vi "Get MetaData from Configurations.vi"(8 "error in":errorcluster, 10 "Measurement":refnum<class "MeasurementService.lvclass">, 11 "Configuration Cluster":variant) -> (0 "error out":errorcluster, 3 "configuration_parameters":T1[](array[typedef]))   [LabVIEW 2020, in "MeasurementLink Measurement Server.lvlib"]
uses:
  MeasurementLink Measurement Server.lvlib
  MeasurementLink Measurement Server Internal/RPC Messages/ni_measurementlink_measurement_v1_ConfigurationParameter.ctl
  MeasurementLink Measurement Server Internal/RPC Messages/ni_measurementlink_measurement_v1_ConfigurationParameter_AnnotationsEntry.ctl
  <vilib>/Utility/Data Type/NI_Data Type.lvlib
  MeasurementLink Measurement Server Internal/MeasurementLink Measurement Server Internal.lvlib
  RPC Service/MeasurementService/MeasurementService.lvclass
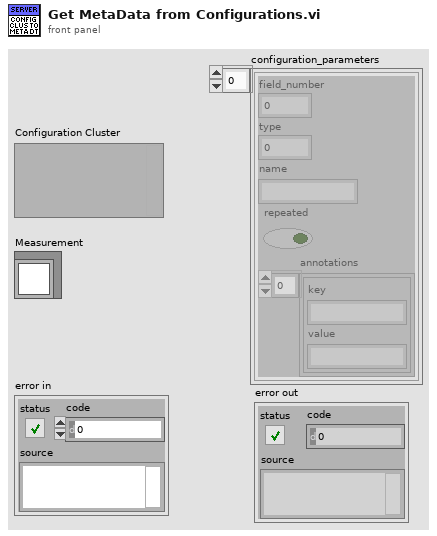
[diagram p1: front panel]
types:
  T1 = typedef "MeasurementLink Measurement Server Internal.lvlib/ni_measurementlink_measurement_v1_ConfigurationParameter.ctl" = cluster{"field_number":i32, "type":i32, "name":string, "repeated":bool, "annotations":T2[]}
  T2 = typedef "MeasurementLink Measurement Server Internal.lvlib/ni_measurementlink_measurement_v1_ConfigurationParameter_AnnotationsEntry.ctl" = cluster{"key":string, "value":string}
  T3 = cluster{"Parameter Name":string, "Annotations":cluster{"key":string, "value":string}[]}[]
  T4 = typedef "NI_Data Type.lvlib/Data Type.ctl" = enum8{"Invalid Type", "Void", "I8", "I16", "I32", "I64", "U8", "U16", "U32", "U64", "Single Float", "Double Float", "Extended Float", "Single Complex", "Double Complex", "Extended Complex", "Enum U8", "Enum U16", "Enum U32", "Enum U64", "Single Float With Unit", "Double Float With Unit", "Extended Float With Unit", "Single Complex with Unit", "Double Complex with Unit", "Extended Complex with Unit", "Boolean", "String", "Path", "Picture", "Tag", "Array", "Cluster", "Variant", "LV Variant", "Waveform", "Timestamp", "Digital Waveform", "Digital Data", "ExpressData", "Refnum", "External Data", "VI", "Poly VI", "LabVIEW Class Instance", "Fixed Point", "Set Collection", "Map Collection"}
  T5 = typedef "MeasurementLink Measurement Server.lvlib/google_protobuf_Field_Kind.ctl" = enum32{"TYPE_UNKNOWN", "TYPE_DOUBLE", "TYPE_FLOAT", "TYPE_INT64", "TYPE_UINT64", "TYPE_INT32", "TYPE_FIXED64", "TYPE_FIXED32", "TYPE_BOOL", "TYPE_STRING", "TYPE_GROUP", "TYPE_MESSAGE", "TYPE_BYTES", "TYPE_UINT32", "TYPE_ENUM", "TYPE_SFIXED32", "TYPE_SFIXED64", "TYPE_SINT32", "TYPE_SINT64"}
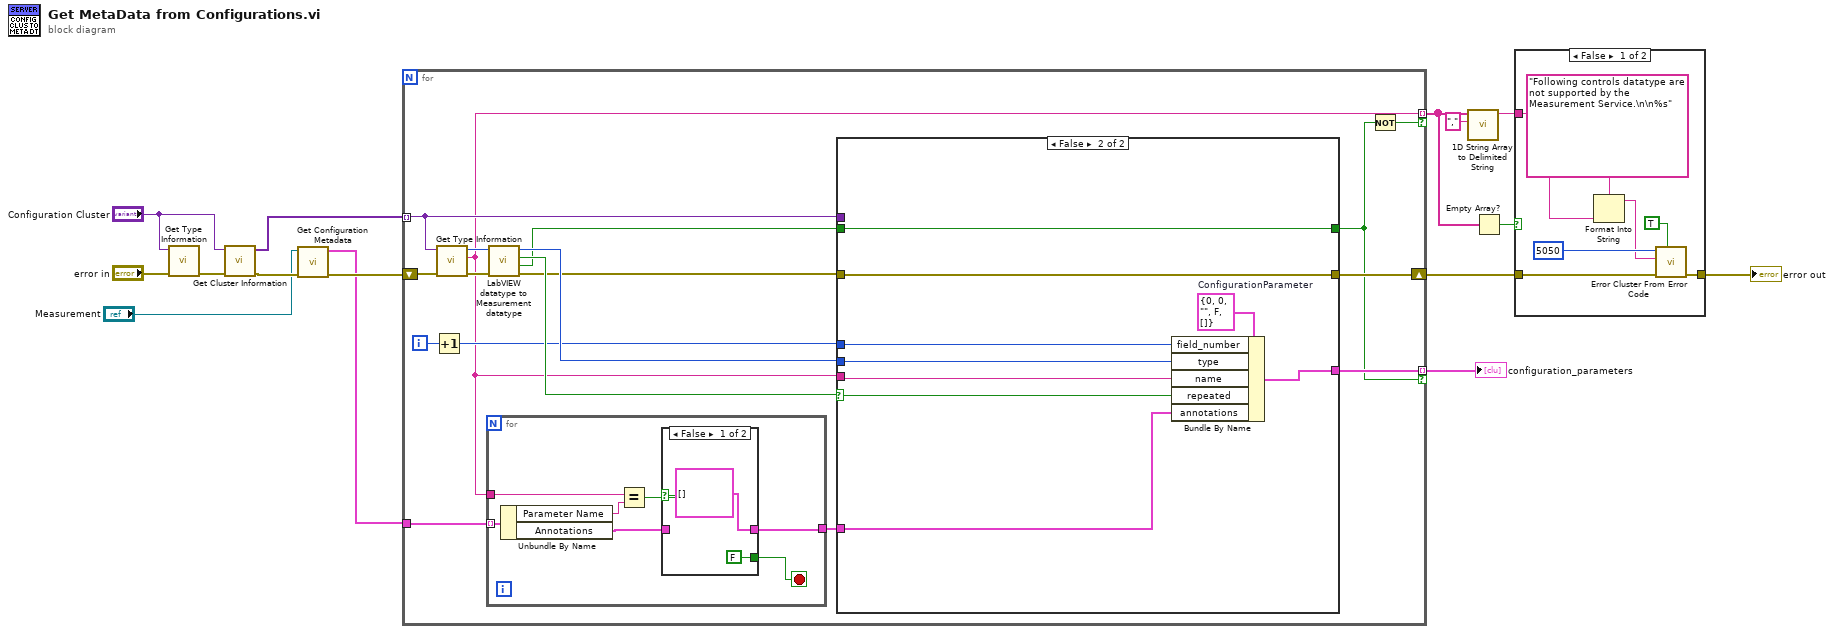
[diagram p0: block diagram]
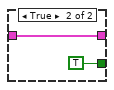
[diagram p3: hidden frame]
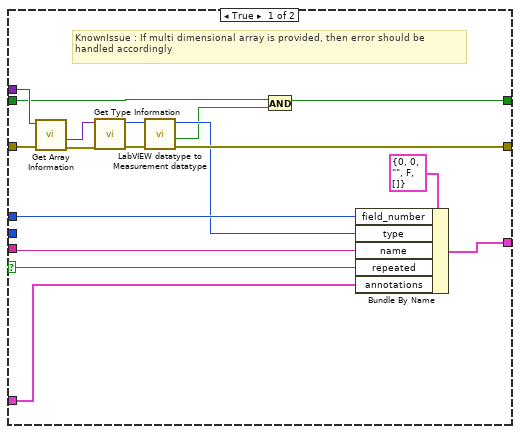
[diagram p4: hidden frame]
diagram:
  n1 = call <vilib>:"Get Type Information.vi"("error in (no error)"="error in", "variant"="Configuration Cluster") -> ("error out"=w15:errorcluster)  [unwired: 5 in, 4 out]
  n2 = call <vilib>:"Get Cluster Information.vi"("error in (no error)"=w15, "variant"="Configuration Cluster") -> ("error out"=w4:errorcluster, "cluster elements"=w14:variant[])  [unwired: 8 in]
  n3 = call "Get Configuration Metadata.vi"("error in (no error)"=w4, "Measurement"="Measurement") -> ("error out"=w3:errorcluster, "Metadata Value"=w2:T3)  [unwired: 8 in]
  n4 = for {
    tunnel: w14 -> [w26] mode=indexing
    tunnel: [w27] -> w13 mode=indexing if=w20
    shift-right: [w22] -> w11
    shift-left: w3 -> [w32]
    tunnel: [w17] -> w10 mode=indexing if=w19
    tunnel: w2 -> [w18]
    i -> [w31]
    n5 = Increment(x=w31) -> (x+1=w23:i32)
    n6 = call <vilib>:"Get Type Information.vi"("error in (no error)"=w32, "variant"=w26) -> ("error out"=w25:errorcluster, "name"=w17:string, "type"=w30:T4)  [unwired: 5 in, 2 out]
    n7 = for {
      tunnel: w18 -> [w38] mode=indexing
      tunnel: w17 -> [w39]
      tunnel: [w34] -> w16
      stop <- w33 stop-if-true
      n8 = Unbundle By Name(w38) -> ("Parameter Name"=w37:string, "Annotations"=w35:cluster{"key":string, "value":string}[])
      n9 = Equal?(x=w39, y=w37) -> (x = y?=w36:bool)
      n10 = case shown="False" w36 {
        tunnel: w35 -> [_ w43]
        tunnel: [cluster{"key":string, "value":string}[] [] ("Annotations") w43] -> w34
        tunnel: [FALSE TRUE] -> w33
        frame False {
        }
        frame True {
        }
      }
    }
    n11 = call "LabVIEW datatype to Measurement datatype.vi"("error in"=w25, "type"=w30) -> ("error out"=w24:errorcluster, "Supported?"=w21:bool, "Array?"=w28:bool, "MessageElementType"=w29:T5)  [unwired: 6 in]
    n12 = case shown="False" w28 {
      selector: w28 -> [w60 w69]
      tunnel: w23 -> [w50 w65]
      tunnel: w29 -> [_ w63]
      tunnel: [w59 w68] -> w27
      tunnel: w24 -> [w58 w67]
      tunnel: w26 -> [w57 _]
      tunnel: [w53 w67] -> w22
      tunnel: w17 -> [w48 w64]
      tunnel: w21 -> [w47 w62]
      tunnel: [w46 w62] -> w20
      tunnel: w16 -> [w44 w61]
      frame True {
        # "KnownIssue : If multi dimensional array is provided, then error should be handled accordingly"
        n13 = call <vilib>:"Get Array Information.vi"("error in (no error)"=w58, "variant"=w57) -> ("error out"=w56:errorcluster, "array element data type"=w52:variant)  [unwired: 6 in, 2 out]
        n14 = call <vilib>:"Get Type Information.vi"("error in (no error)"=w56, "variant"=w52) -> ("error out"=w54:errorcluster, "type"=w55:T4)  [unwired: 5 in, 3 out]
        n15 = call "LabVIEW datatype to Measurement datatype.vi"("error in"=w54, "type"=w55) -> ("error out"=w53:errorcluster, "Supported?"=w45:bool, "MessageElementType"=w49:T5)  [unwired: 6 in, 1 out]
        n16 = And(x=w47, y=w45) -> (x .and. y?=w46:bool)
        n17 = Bundle By Name(cluster=T1 {"field_number"=0, "type"=0, "name"="", "repeated"=FALSE, "annotations"=[]} ("ConfigurationParameter"), "field_number"=w50, "type"=w49, "name"=w48, "repeated"=w60, "annotations"=w44) -> (w59:T1)
      }
      frame False {
        w66 = T1 {"field_number"=0, "type"=0, "name"="", "repeated"=FALSE, "annotations"=[]}  # ConfigurationParameter
        n18 = Bundle By Name(cluster=w66, "field_number"=w65, "type"=w63, "name"=w64, "repeated"=w69, "annotations"=w61) -> (w68:T1)
      }
    }
    n19 = Not(x=w20) -> (.not. x?=w19:bool)
  }
  "configuration_parameters" <- w13
  n20 = call <vilib>:"1D String Array to Delimited String.vi"("delimiter"=",", "string array"=w10) -> ("delimited string"=w8:string)  [unwired: 9 in]
  n21 = Empty Array?(array=w10) -> (empty?=w9:bool)
  n22 = case shown="False" w9 {
    tunnel: w11 -> [w76 w77]
    tunnel: [w75 w77] -> w5
    tunnel: w8 -> [w72 _]
    frame False {
      n23 = Format Into String(format string="Following controls datatype are not supported by the Measurement Service.\n\n%s", w72) -> (resulting string=w71:string)  [unwired: 2 in, 1 out]
      n24 = call <vilib>:"Error Cluster From Error Code.vi"("show call chain? (False)"=TRUE, "error in (no error)"=w76, "error message (\"\")"=w71, "error code (0)"=5050) -> ("error out"=w75:errorcluster)  [unwired: 5 in]
    }
    frame True {
    }
  }
  "error out" <- w5
